vi "Read GlobalBlockSize.vi"(8 "error in (no error)":errorcluster, 11 "ChassisCfg in":refnum<class "ChassisCfg.lvclass">) -> (0 "error out":errorcluster, 2 "LockToLS":T1, 3 "ChassisCfg out":refnum<class "ChassisCfg.lvclass">)   [LabVIEW 2012, in "Configuration Grandmaster.lvlib" / "ChassisCfg.lvclass"]
uses:
  ChassisCfg.lvclass
  Common/Controls/LS Lock Sizes.ctl
  ChassisCfg.lvclass/ChassisCfg.ctl
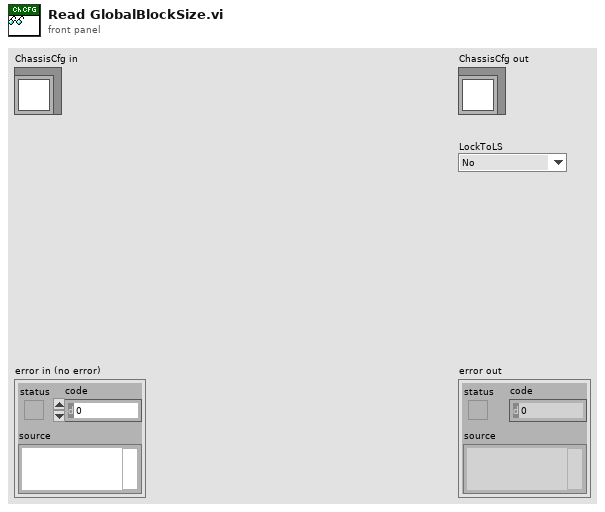
[diagram p1: front panel]
types:
  T1 = typedef "LS Lock Sizes.ctl" = enum16{"No", "250ms", "500ms", "1s"}
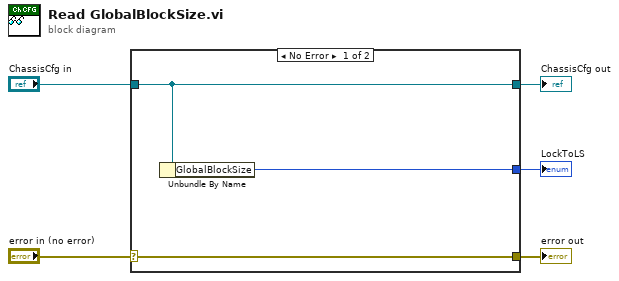
[diagram p0: block diagram]
diagram:
  n1 = case shown="No Error" "error in (no error)" {
    selector: "error in (no error)" -> [w8 w9]
    tunnel: [w8 w9] -> w4
    tunnel: [w7 w10] -> w2
    tunnel: "ChassisCfg in" -> [w7 w10]
    tunnel: [w6 _] -> w1
    frame No Error {
      n2 = Unbundle By Name(w7) -> ("GlobalBlockSize"=w6:T1)
    }
    frame Error {
    }
  }
  "error out" <- w4
  "ChassisCfg out" <- w2
  "LockToLS" <- w1
